vi "test_SCD_Setup_Testenvironment.vi"(6 "Delay between send and receive [ms]":i32=100, 8 "error in":errorcluster) -> (0 "error out":errorcluster, 2 "device open for communication?":bool, 3 "SCD out":refnum<class "SCD.lvclass">)   [LabVIEW 2023]
uses:
  Classes/DeviceManager/DeviceManager.lvlib
  <userlib>/_OpenG.lib/error/error.llb/openg_error.lvlib
  Classes/SCD/SCD.lvclass
panel:
  # "Connector Pane"
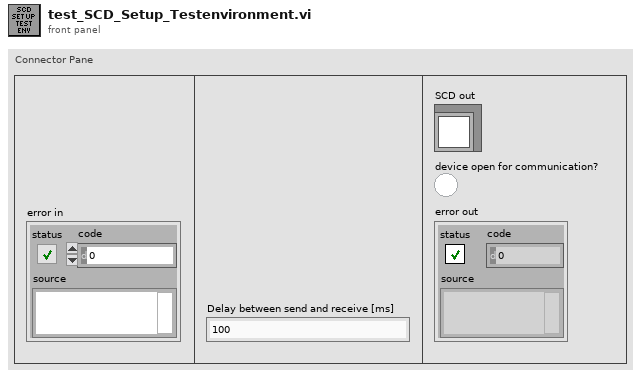
[diagram p1: front panel]
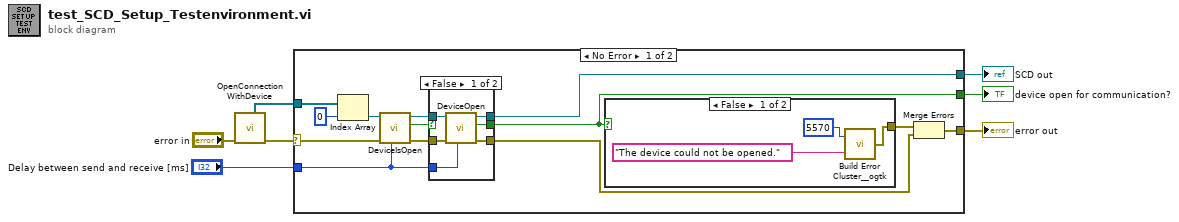
[diagram p0: block diagram]
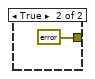
[diagram p3: hidden frame]
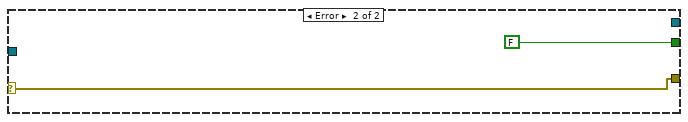
[diagram p4: hidden frame]
diagram:
  n1 = call "OpenConnectionWithDevice.vi"("error in"="error in") -> ("error out"=w3:errorcluster, "SCDs"=w2:refnum<class "SCD.lvclass">[])  [unwired: 6 in, 3 out]
  n2 = case shown="No Error" w3 {
    selector: w3 -> [w12 w35]
    tunnel: [w19 w35] -> w6
    tunnel: [w9 FALSE ("CCD open for communication?")] -> w5
    tunnel: [w11 _] -> w4
    tunnel: w2 -> [w17 _]
    tunnel: "Delay between send and receive [ms]" -> [w8 _]
    frame No Error {
      n3 = Index Array(array=w17, index=0) -> (element=w13:refnum<class "SCD.lvclass">)
      n4 = call-dynamic "DeviceIsOpen.vi"("Delay between send and receive [ms]"=w8, "error in (no error)"=w12, "SCD in"=w13) -> ("error out"=w14:errorcluster, "device is open?"=w15:bool, "SCD out"=w16:refnum<class "SCD.lvclass">)  [unwired: 5 in, 1 out]
      n5 = case shown="False" w15 {
        selector: w15 -> [_ w27]
        tunnel: [w26 w27] -> w9
        tunnel: [w25 w28] -> w10
        tunnel: [w24 w29] -> w11
        tunnel: w14 -> [w23 w28]
        tunnel: w16 -> [w22 w29]
        tunnel: w8 -> [w21 _]
        frame False {
          n6 = call-dynamic "DeviceOpen.vi"("Delay between send and receive [ms]"=w21, "error in (no error)"=w23, "SCD in"=w22) -> ("error out"=w25:errorcluster, "device is open?"=w26:bool, "SCD out"=w24:refnum<class "SCD.lvclass">)  [unwired: 5 in, 1 out]
        }
        frame True {
        }
      }
      n7 = case shown="False" w9 {
        tunnel: [w31 errorcluster {"status"=FALSE, "code"=0, "source"=""} ("error in 2")] -> w18
        frame False {
          n8 = call <userlib>:"Build Error Cluster__ogtk.vi"("String to Prepend to source (\"\")"="The device could not be opened." ("String to Prepend to source (\"\")"), "code"=5570) -> ("error out"=w31:errorcluster)
        }
        frame True {
        }
      }
      n9 = Merge Errors(w18, w10) -> (w19:errorcluster)
    }
    frame Error {
    }
  }
  "error out" <- w6
  "device open for communication?" <- w5
  "SCD out" <- w4
